vi "Write-on-FPElement.vi"(8 "error in (no error)":errorcluster, 9 "Data type in":string, 10 "Value in":string, 11 "Control in":refnum<vi>) -> (0 "error out":errorcluster, 1 "Data type out":string, 2 "Value out":string, 3 "Control out":refnum<vi>)   [LabVIEW 2016]
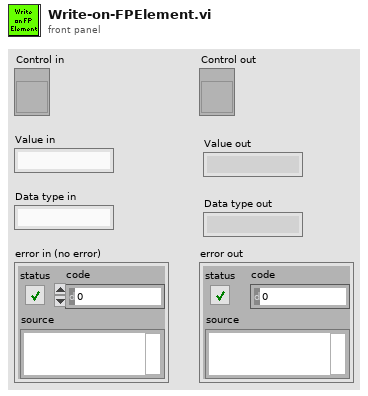
[diagram p1: front panel]
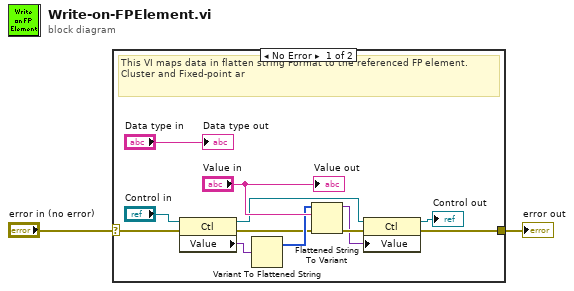
[diagram p0: block diagram]
diagram:
  n1 = case shown="No Error" "error in (no error)" {
    selector: "error in (no error)" -> [w11 w15]
    tunnel: [w14 w15] -> w2
    frame No Error {
      # "This VI maps data in flatten string Format to the referenced FP element.\nCluster and Fixed-point ar"
      n2 = property class="Ctl"(reference="Control in", error in=w11) -> (reference out=w6:refnum<vi>, error out=w3:errorcluster, "Value"=w5:variant)
      n3 = Variant To Flattened String(Variant=w5) -> (1:w4:i16[])  [unwired: 1 out]
      n4 = Flattened String To Variant(4:w3, 6:"Value in", 7:w4) -> (0:w10:errorcluster, 3:w8:variant)
      n5 = property class="Ctl"(reference=w6, error in=w10, "Value"=w8) -> (reference out=→"Control out":refnum<vi>, error out=w14:errorcluster)
      "Data type out" <- "Data type in"
      "Value out" <- "Value in"
    }
    frame Error {
    }
  }
  "error out" <- w2
